vi "BoolDelay.vi"(10 "Delay":dbl, 11 "Input":bool) -> (3 "Output":bool)   [LabVIEW 2012]
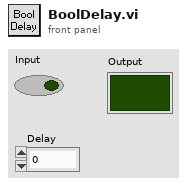
[diagram p1: front panel]
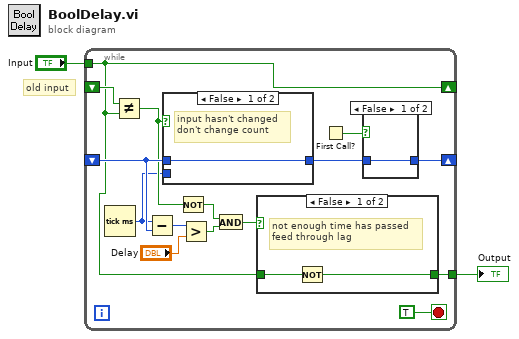
[diagram p0: block diagram]
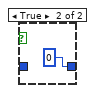
[diagram p2: hidden frame]
diagram:
  # "old input"
  n1 = while {
    tunnel: "Input" -> [w12]
    shift-right: [w12] -> _
    shift-left: _ -> [w16]
    shift-right: [w4] -> _
    shift-left: _ -> [w13]
    tunnel: [w11] -> w1
    stop <- TRUE stop-if-true
    n2 = Tick Count (ms)() -> (millisecond timer value=w6:u32)
    n3 = Not Equal?(x=w16, y=w12) -> (x != y?=w7:bool)
    n4 = Subtract(x=w6, y=w13) -> (x-y=w15:u32)
    n5 = case shown="False" w7 {
      tunnel: [w23 w24] -> w3
      tunnel: w13 -> [w23 _]
      tunnel: w6 -> [_ w24]
      frame False {
        # "input hasn't changed\ndon't change count"
      }
      frame True {
        # "if input changed start\ncounting"
      }
    }
    n6 = Not(x=w7) -> (.not. x?=w8:bool)
    n7 = Greater?(x=w15, y="Delay") -> (0:w9:bool)
    n8 = And(x=w8, y=w9) -> (x .and. y?=w10:bool)
    n9 = case shown="False" w10 {
      tunnel: w12 -> [w21 w22]
      tunnel: [w20 w22] -> w11
      frame False {
        # "not enough time has passed\nfeed through lag"
        n10 = Not(x=w21) -> (.not. x?=w20:bool)
      }
      frame True {
        # "enough time has\npassed feed through\nreal outout"
      }
    }
    n11 = First Call?() -> (First Call?: T/F=w5:bool)
    n12 = case shown="False" w5 {
      tunnel: [w18 0] -> w4
      tunnel: w3 -> [w18 _]
      frame False {
      }
      frame True {
      }
    }
  }
  "Output" <- w1
